vi "Main Tclk.vi"() -> ()   [LabVIEW 2018] (continued)
                                n3267 = local write "SEM Scan Parameters"(w8659) -> ()
                                n3268 = Build Array(w8675, w8670) -> (w8655:T76)
                                n3269 = local write "Auto Aln X"(w8655) -> ()
                              }
                            }
                          }
                          frame #2 {
                            n3270 = Array Size(array=w8677) -> (size(s)=w8680:i32)
                            n3271 = Greater Or Equal?(x=w8680, y=2) -> (x >= y?=w8681:bool)
                            n3272 = Array Subset(array=w8678, length=w8680) -> (w8679:sgl[])  [unwired: 1 in]
                            n3273 = case shown="True" w8681 {
                              tunnel: w8677 -> [_ w8693]
                              tunnel: w8679 -> [_ w8689]
                              tunnel: [_ w8683] -> w8676
                              frame False {
                              }
                              frame True {
                                n3274 = Array Max & Min(array=w8689) -> (max value=w8691:sgl, min value=w8690:sgl)  [unwired: 2 out]
                                n3275 = Array Max & Min(array=w8693) -> (max value=w8695:sgl, min value=w8696:sgl)  [unwired: 2 out]
                                n3276 = Subtract(x=w8691, y=w8690) -> (x-y=w8692:sgl)
                                n3277 = Subtract(x=w8695, y=w8696) -> (x-y=w8694:sgl)
                                n3278 = expression code="x*0.2"(w8692) -> (w8688:sgl)
                                n3279 = expression code="x*0.2"(w8694) -> (w8697:sgl)
                                n3280 = Add(x=w8691, y=w8688) -> (x+y=w8687:sgl)
                                n3281 = Subtract(x=w8690, y=w8688) -> (x-y=w8686:sgl)
                                n3282 = Add(x=w8695, y=w8697) -> (x+y=w8685:sgl)
                                n3283 = Subtract(x=w8696, y=w8697) -> (x-y=w8684:sgl)
                                n3284 = Bundle(w8687, w8686, w8685, w8684) -> (w8683:cluster{sgl, sgl, sgl, sgl})  [unwired: 1 in]
                                n3285 = property on="Auto Aln X" class="XYGraph (strict)"("XScale.Maximum"=w8687, "XScale.Minimum"=w8686, "YScale.Maximum"=w8685, "YScale.Minimum"=w8684) -> ()  [unwired: 2 in, 2 out]
                              }
                            }
                          }
                        }
                      }
                    }
                    n3286 = And Array Elements(Boolean array=w8539) -> (logical AND=w8538:bool)
                    n3287 = local write "AAX Success tiled"(w8541) -> ()
                    n3288 = local write "AAX Graph scales tiled"(w8536) -> ()
                    n3289 = local write "AlnX array tiled"(w8545) -> ()
                    n3290 = local write "AAX Graph tiled"(w8537) -> ()
                    n3291 = local write "Best Aln X FI tiled"(w8543) -> ()
                    n3292 = local write "Skip Steps tiled"(w8544) -> ()
                    n3293 = local write "Best Aln X (%) tiled"(w8542) -> ()
                    n3294 = case shown="True" w8538 {
                      frame False {
                      }
                      frame True {
                        w8557 = T44."Enabled" ("Disabled")
                        w8559 = sgl[][][] [] ("FI array tiled")
                        n3295 = local read "SEM Scan Parameters"() -> (w8556:T26)
                        n3296 = Unbundle By Name(w8556) -> ("Y tiles"=w8552:u8, "X tiles"=w8553:u8)
                        n3297 = local write "AA Count"(u8 0 ("AA Count")) -> ()
                        n3298 = local write "FI array tiled"(w8559) -> ()
                        n3299 = local write "AlnX array tiled"(w8559) -> ()
                        n3300 = local write "Aln Options"(enum16{"Defaut", "Aln X", "Aln Y"}."Aln Y" ("Aln Options")) -> ()
                        n3301 = property on="Auto Align" class="Bool (strict)"("DisabledEnum"=w8557) -> ()  [unwired: 2 in, 2 out]
                        n3302 = property on="AA Steps" class="DigNum (strict)"("DisabledEnum"=w8557) -> ()  [unwired: 2 in, 2 out]
                        n3303 = Initialize Array(u8 0 ("Skip Steps"), w8552, w8553) -> (w8554:u8[][])
                        n3304 = local write "Skip Steps tiled"(w8554) -> ()
                      }
                    }
                  }
                  frame True {
                  }
                }
              }
              frame #35 {
                n3305 = local read "AlnY array tiled"() -> (w8699:sgl[][][])
                n3306 = local read "FI array tiled"() -> (w8700:sgl[][][])
                n3307 = local read "AA Count"() -> (w8701:u8)
                n3308 = local read "AA Steps"() -> (w8703:u8)
                n3309 = local read "Skip Steps tiled"() -> (w8702:u8[][])
                n3310 = local read "Auto Align"() -> (w8704:bool)
                n3311 = Empty Array?(array=w8699) -> (empty?=w8698:bool)
                n3312 = Not(x=w8704) -> (.not. x?=w8705:bool)
                n3313 = case shown="False" w8698 {
                  tunnel: w8699 -> [w8720 _]
                  tunnel: w8700 -> [w8719 _]
                  tunnel: w8701 -> [w8718 _]
                  tunnel: w8702 -> [w8717 _]
                  tunnel: w8703 -> [w8716 _]
                  tunnel: w8705 -> [w8710 _]
                  frame False {
                    n3314 = for {
                      tunnel: w8720 -> [w8741] mode=indexing
                      tunnel: w8719 -> [w8740] mode=indexing
                      tunnel: w8718 -> [w8739]
                      tunnel: w8717 -> [w8738] mode=indexing
                      tunnel: w8716 -> [w8737]
                      tunnel: [w8736] -> w8715 mode=indexing
                      tunnel: [w8734] -> w8714 mode=indexing
                      tunnel: [w8733] -> w8713 mode=indexing
                      tunnel: [w8732] -> w8712 mode=indexing
                      tunnel: [w8731] -> w8711 mode=indexing
                      tunnel: w8710 -> [w8730]
                      tunnel: [w8729] -> w8709 mode=indexing
                      tunnel: [w8728] -> w8707 mode=indexing
                      tunnel: [w8727] -> w8706 mode=indexing
                      i -> [w8735]
                      n3315 = for {
                        tunnel: w8741 -> [w8757] mode=indexing
                        tunnel: w8740 -> [w8756] mode=indexing
                        tunnel: w8739 -> [w8755]
                        tunnel: w8738 -> [w8754] mode=indexing
                        tunnel: w8737 -> [w8753]
                        tunnel: [w8752] -> w8736 mode=indexing
                        tunnel: w8735 -> [w8751]
                        tunnel: [w8749] -> w8734 mode=indexing
                        tunnel: [w8748] -> w8733 mode=indexing
                        tunnel: [w8747] -> w8732 mode=indexing
                        tunnel: [w8746] -> w8731 mode=indexing
                        tunnel: w8730 -> [w8745]
                        tunnel: [w8744] -> w8729 mode=indexing
                        tunnel: [w8743] -> w8728 mode=indexing
                        tunnel: [w8742] -> w8727 mode=indexing
                        i -> [w8750]
                        n3316 = stacked-sequence {
                          seq-local: [w8760 _ _] -> [_ w8798 _]
                          seq-local: [w8758 _ _] -> [_ w8789 _]
                          tunnel: w8757 -> [w8765 w8790 w8845]
                          tunnel: w8756 -> [w8764 w8803 w8844]
                          tunnel: w8755 -> [w8762 w8786 _]
                          tunnel: w8754 -> [w8759 _ _]
                          tunnel: w8753 -> [w8761 w8787 _]
                          tunnel: [_ w8799 _] -> w8752
                          tunnel: w8751 -> [_ w8797 _]
                          tunnel: w8750 -> [_ w8796 _]
                          tunnel: [w8758 _ _] -> w8749
                          tunnel: [_ w8795 _] -> w8748
                          tunnel: [_ w8794 _] -> w8747
                          tunnel: [_ w8793 _] -> w8746
                          tunnel: w8745 -> [_ w8792 _]
                          tunnel: [_ w8791 _] -> w8744
                          tunnel: [_ w8788 _] -> w8743
                          tunnel: [_ _ w8843] -> w8742
                          frame #0 {
                            n3317 = Subtract(x=w8761, y=w8759) -> (x-y=w8763:u8)
                            n3318 = Less?(x=w8762, y=w8763) -> (x < y?=w8766:bool)
                            n3319 = case shown="True" w8766 {
                              tunnel: w8765 -> [w8768 w8773]
                              tunnel: w8762 -> [_ w8772]
                              tunnel: w8764 -> [_ w8774]
                              tunnel: [w8768 w8771] -> w8760
                              tunnel: w8759 -> [w8767 w8770]
                              tunnel: [w8767 w8769] -> w8758
                              frame False {
                              }
                              frame True {
                                n3320 = Index Array(array=w8773, index=w8772) -> (element=w8776:sgl)
                                n3321 = call "1D Parabolic Max.vi"("Y"=w8774, "Xt"=w8776, "X"=w8773) -> ("Y(Xt) < Ymin"=w8775:bool)  [unwired: 1 in, 7 out]
                                n3322 = case shown="True" w8775 {
                                tunnel: w8772 -> [_ w8782]
                                tunnel: w8773 -> [w8778 w8783]
                                tunnel: w8770 -> [w8777 w8780]
                                tunnel: [w8778 w8781] -> w8771
                                tunnel: [w8777 w8779] -> w8769
                                frame False {
                                }
                                frame True {
                                n3323 = Delete From Array(array=w8783, length=1, index=w8782) -> (array with subset deleted=w8781:sgl[])  [unwired: 1 out]
                                n3324 = Increment(x=w8780) -> (x+1=w8779:u8)
                                }
                                }
                              }
                            }
                          }
                          frame #1 {
                            n3325 = Subtract(x=w8787, y=w8789) -> (x-y=w8802:u8)
                            n3326 = call "1D Parabolic Max.vi"("Y"=w8803, "X"=w8790) -> ("Found max"=w8793:bool, "Ymax"=w8800:dbl, "Xmax"=w8804:dbl, "Finer Best Polynomial Fit"=w8806:dbl[], "Finer X"=w8801:dbl[])  [unwired: 2 in, 3 out]
                            n3327 = Greater Or Equal?(x=w8786, y=w8802) -> (x >= y?=w8805:bool)
                            n3328 = Subtract(x=w8787, y=w8786) -> (x-y=w8785:u8)
                            n3329 = Compound Arithmetic op=OR(w8793, w8805, w8792) -> (w8791:bool)
                            n3330 = case shown="True" w8791 {
                              tunnel: w8804 -> [_ w8824]
                              tunnel: w8803 -> [w8808 w8836]
                              tunnel: w8798 -> [w8816 _]
                              tunnel: w8806 -> [_ w8835]
                              tunnel: w8801 -> [_ w8834]
                              tunnel: w8800 -> [_ w8825]
                              tunnel: w8785 -> [_ w8833]
                              tunnel: w8786 -> [_ w8831]
                              tunnel: [w8816 w8830] -> w8799
                              tunnel: w8797 -> [w8813 w8821]
                              tunnel: w8796 -> [w8814 w8820]
                              tunnel: [w8807 w8825] -> w8795
                              tunnel: [w8810 w8824] -> w8794
                              tunnel: w8790 -> [w8811 w8823]
                              tunnel: [w8815 w8822] -> w8788
                              frame False {
                                n3331 = Build Cluster Array(w8811, w8808) -> (w8817:cluster{"Center":sgl, "A Img Focus Index":sgl}[])
                                n3332 = Sort 1D Array(array=w8817) -> (sorted array=w8818:cluster{"Center":sgl, "A Img Focus Index":sgl}[])
                                n3333 = Bundle(w8818) -> (w8819:T74)  [unwired: 1 in]
                                n3334 = Build Array(w8819) -> (w8815:T75)
                                n3335 = local write "AAY Y tile"(w8813) -> ()
                                n3336 = local write "AAY X tile"(w8814) -> ()
                                n3337 = local write "Auto Aln Y"(w8815) -> ()
                                n3338 = Index Array(array=w8811, index=0) -> (element=w8810:sgl)
                                n3339 = Index Array(array=w8808, index=0) -> (element=w8807:sgl)
                              }
                              frame True {
                                n3340 = local read "SEM Scan Parameters"() -> (w8828:T26)
                                n3341 = Initialize Array(w8824, w8833) -> (w8832:dbl[])
                                n3342 = Replace Array Subset(array=w8823, new element=w8832, index=w8831) -> (w8830:sgl[])
                                n3343 = Build Cluster Array(w8823, w8836) -> (w8841:cluster{"Center":sgl, "A Img Focus Index":sgl}[])
                                n3344 = Build Cluster Array(w8834, w8835) -> (w8838:cluster{dbl, dbl}[])
                                n3345 = local write "AAY Y tile"(w8821) -> ()
                                n3346 = local write "AAY X tile"(w8820) -> ()
                                n3347 = Unbundle By Name(w8828) -> ("Y aln"=w8829:sgl[][])
                                n3348 = Sort 1D Array(array=w8841) -> (sorted array=w8840:cluster{"Center":sgl, "A Img Focus Index":sgl}[])
                                n3349 = Sort 1D Array(array=w8838) -> (sorted array=w8839:cluster{dbl, dbl}[])
                                n3350 = Replace Array Subset(array=w8829, new element=w8824, index (row)=w8821, index (col)=w8820) -> (w8827:sgl[][])
                                n3351 = Bundle(w8840) -> (w8842:T74)  [unwired: 1 in]
                                n3352 = Bundle(w8839) -> (w8837:cluster{cluster{dbl, dbl}[]})  [unwired: 1 in]
                                n3353 = Bundle By Name(cluster=w8828, "Y aln"=w8827) -> (w8826:T26)
                                n3354 = local write "SEM Scan Parameters"(w8826) -> ()
                                n3355 = Build Array(w8842, w8837) -> (w8822:T76)
                                n3356 = local write "Auto Aln Y"(w8822) -> ()
                              }
                            }
                          }
                          frame #2 {
                            n3357 = Array Size(array=w8844) -> (size(s)=w8847:i32)
                            n3358 = Greater Or Equal?(x=w8847, y=2) -> (x >= y?=w8848:bool)
                            n3359 = Array Subset(array=w8845, length=w8847) -> (w8846:sgl[])  [unwired: 1 in]
                            n3360 = case shown="True" w8848 {
                              tunnel: w8844 -> [_ w8860]
                              tunnel: w8846 -> [_ w8856]
                              tunnel: [_ w8850] -> w8843
                              frame False {
                              }
                              frame True {
                                n3361 = Array Max & Min(array=w8856) -> (max value=w8858:sgl, min value=w8857:sgl)  [unwired: 2 out]
                                n3362 = Array Max & Min(array=w8860) -> (max value=w8862:sgl, min value=w8863:sgl)  [unwired: 2 out]
                                n3363 = Subtract(x=w8858, y=w8857) -> (x-y=w8859:sgl)
                                n3364 = Subtract(x=w8862, y=w8863) -> (x-y=w8861:sgl)
                                n3365 = expression code="x*0.2"(w8859) -> (w8855:sgl)
                                n3366 = expression code="x*0.2"(w8861) -> (w8864:sgl)
                                n3367 = Add(x=w8858, y=w8855) -> (x+y=w8854:sgl)
                                n3368 = Subtract(x=w8857, y=w8855) -> (x-y=w8853:sgl)
                                n3369 = Add(x=w8862, y=w8864) -> (x+y=w8852:sgl)
                                n3370 = Subtract(x=w8863, y=w8864) -> (x-y=w8851:sgl)
                                n3371 = Bundle(w8854, w8853, w8852, w8851) -> (w8850:cluster{sgl, sgl, sgl, sgl})  [unwired: 1 in]
                                n3372 = property on="Auto Aln Y" class="XYGraph (strict)"("XScale.Maximum"=w8854, "XScale.Minimum"=w8853, "YScale.Maximum"=w8852, "YScale.Minimum"=w8851) -> ()  [unwired: 2 in, 2 out]
                              }
                            }
                          }
                        }
                      }
                    }
                    n3373 = And Array Elements(Boolean array=w8709) -> (logical AND=w8708:bool)
                    n3374 = local write "AAY Success tiled"(w8711) -> ()
                    n3375 = local write "AAY Graph scales tiled"(w8706) -> ()
                    n3376 = local write "AlnY array tiled"(w8715) -> ()
                    n3377 = local write "AAY Graph tiled"(w8707) -> ()
                    n3378 = local write "Best Aln Y FI tiled"(w8713) -> ()
                    n3379 = local write "Skip Steps tiled"(w8714) -> ()
                    n3380 = local write "Best Aln Y (%) tiled"(w8712) -> ()
                    n3381 = case shown="True" w8708 {
                      frame False {
                      }
                      frame True {
                        w8723 = T44."Enabled" ("Disabled")
                        w8725 = sgl[][][] [] ("FI array tiled")
                        n3382 = local write "Auto Align"(FALSE ("Auto Stig")) -> ()
                        n3383 = local write "AA Count"(u8 0 ("AA Count")) -> ()
                        n3384 = local write "Skip Steps tiled"(u8[][] [] ("AS Count tiled")) -> ()
                        n3385 = local write "FI array tiled"(w8725) -> ()
                        n3386 = local write "AlnX array tiled"(w8725) -> ()
                        n3387 = local write "Aln Options"(enum16{"Defaut", "Aln X", "Aln Y"}."Defaut" ("Aln Options")) -> ()
                        n3388 = property on="Auto Focus" class="Bool (strict)"("DisabledEnum"=w8723) -> ()  [unwired: 2 in, 2 out]
                        n3389 = property on="Auto Stig" class="Bool (strict)"("DisabledEnum"=w8723) -> ()  [unwired: 2 in, 2 out]
                        n3390 = property on="Auto Align" class="Bool (strict)"("DisabledEnum"=w8723) -> ()  [unwired: 2 in, 2 out]
                        n3391 = property on="AA Steps" class="DigNum (strict)"("DisabledEnum"=w8723) -> ()  [unwired: 2 in, 2 out]
                      }
                    }
                  }
                  frame True {
                  }
                }
              }
              frame #36 {
                n3392 = local read "Low Mag SEM"() -> (w8865:T30)
                n3393 = local read "Mid Mag SEM"() -> (w8866:T29)
                n3394 = Unbundle By Name(w8865) -> ("Low mag scan"=w8867:bool)
                n3395 = Unbundle By Name(w8866) -> ("Mid mag scan"=w8868:bool)
                n3396 = case shown="True" w8867 {
                  tunnel: w8865 -> [_ w8891]
                  frame False {
                  }
                  frame True {
                    w8887 = sgl[] [0.0] ("dX (um)")
                    w8888 = u8 1 ("X tiles")
                    w8892 = 0.0 ("X center")
                    n3397 = Unbundle By Name(w8891) -> ("Low mag scan FOV (micron)"=w8889:dbl, "Low mag scan rate (Hz)"=w8901:u32)
                    n3398 = local read "SEM Scan Parameters"() -> (w8894:T26)
                    n3399 = Unbundle By Name(w8894) -> ("Scan rate (Hz)"=w8896:u32, "Oversampling"=w8895:u32)
                    n3400 = expression code="x*1000"(w8889) -> (w8902:dbl)
                    n3401 = Multiply(x=w8896, y=w8895) -> (x*y=w8897:u32)
                    n3402 = Divide(x=w8897, y=w8901) -> (x/y=w8898:dbl)
                    n3403 = Divide(x=w8902, y=u32 512 ("X resolution")) -> (x/y=w8900:dbl)
                    n3404 = Bundle By Name(cluster=w8894, "X size (um)"=w8889, "Y size (um)"=w8889, "X center (um)"=w8892, "Y center (um)"=w8892, "X size (V)"=20.0, "Scan rate (Hz)"=w8901, "Oversampling"=w8898, "X tiles"=w8888, "Y tiles"=w8888, "Frames"=w8888, "dX (um)"=w8887, "dY (um)"=w8887, "Pixel size (nm)"=w8900) -> (w8890:T26)
                    n3405 = local write "SEM Low Mag Scan Parameters"(w8890) -> ()
                  }
                }
                n3406 = case shown="True" w8868 {
                  tunnel: w8866 -> [_ w8875]
                  frame False {
                  }
                  frame True {
                    w8869 = sgl[] [0.0] ("dX (um)")
                    w8870 = u8 1 ("X tiles")
                    n3407 = Unbundle By Name(w8875) -> ("X size (um)"=w8881:sgl, "Y size (um)"=w8880:sgl, "X center (um)"=w8879:dbl, "Y center (um)"=w8878:dbl, "Mid mag scan rate (Hz)"=w8877:u32, "Pixel size (nm)"=w8876:sgl)
                    n3408 = local read "SEM Mid Mag Scan Parameters"() -> (w8873:T5)
                    n3409 = local read "SEM Scan Parameters"() -> (w8882:T26)
                    n3410 = Unbundle By Name(w8882) -> ("Scan rate (Hz)"=w8884:u32, "Oversampling"=w8883:u32)
                    n3411 = Unbundle By Name(w8873) -> ("X size (V)"=w8872:dbl)
                    n3412 = Multiply(x=w8884, y=w8883) -> (x*y=w8885:u32)
                    n3413 = Divide(x=w8885, y=w8877) -> (x/y=w8886:dbl)
                    n3414 = Bundle By Name(cluster=w8882, "X size (um)"=w8881, "Y size (um)"=w8880, "X center (um)"=w8879, "Y center (um)"=w8878, "Oversampling auto"=TRUE ("X size auto"), "Scan rate (Hz)"=w8877, "Oversampling"=w8886, "Pixel size (nm)"=w8876, "X size (V)"=w8872, "X tiles"=w8870, "Y tiles"=w8870, "Frames"=w8870, "dX (um)"=w8869, "dY (um)"=w8869) -> (w8871:T26)
                    n3415 = local write "SEM Mid Mag Scan Parameters"(w8871) -> ()
                  }
                }
              }
              frame #37 {
                n3416 = local read "Mid Mag SEM"() -> (w8917:T29)
                n3417 = local read "FIB slice #"() -> (w8911:u32)
                n3418 = Unbundle By Name(w8917) -> ("Mid mag scan"=w8918:bool, "Prior to main scan"=w8919:bool, "Mid mag interval"=w8905:u32)
                n3419 = Equal?(x=u32 1 ("y"), y=w8905) -> (x = y?=w8909:bool)
                n3420 = case shown="False" w8909 {
                  tunnel: [w8923 w8926] -> w8907
                  tunnel: [w8922 w8926] -> w8908
                  tunnel: [w8920 w8926] -> w8906
                  frame False {
                    n3421 = local read "Auto Focus"() -> (w8925:bool)
                    n3422 = local read "Auto Stig"() -> (w8924:bool)
                    n3423 = local read "Auto Align"() -> (w8921:bool)
                    n3424 = Not(x=w8925) -> (.not. x?=w8922:bool)
                    n3425 = Not(x=w8924) -> (.not. x?=w8923:bool)
                    n3426 = Not(x=w8921) -> (.not. x?=w8920:bool)
                  }
                  frame True {
                    w8926 = TRUE
                  }
                }
                n3427 = Subtract(x=w8911, y=u32 2) -> (x-y=w8903:u32)
                n3428 = Quotient & Remainder(x=w8903, y=w8905) -> (x-y*floor(x/y)=w8915:u32)  [unwired: 1 out]
                n3429 = local read "FIB"() -> (w8912:bool)
                n3430 = Not(x=w8919) -> (.not. x?=w8914:bool)
                n3431 = Equal To 0?(x=w8915) -> (x = 0?=w8916:bool)
                n3432 = Compound Arithmetic op=AND(w8912, w8908, w8907, w8906, w8918, w8914, w8916) -> (w8913:bool)
                n3433 = case shown="True" w8913 {
                  frame False {
                    n3434 = local write "Mid Mag SEM on"(FALSE ("Mid Mag SEM on")) -> ()
                    n3435 = local write "MM overhead"(u32 0 ("MM overhead")) -> ()
                  }
                  frame True {
                    w8938 = FALSE ("GetInfo")
                    n3436 = local read "Tiled scan inputs"() -> (w8937:T6)
                    n3437 = local read "SEM Mid Mag Scan Parameters"() -> (w8935:T5)
                    n3438 = local read "File Information"() -> (w8934:T31)
                    n3439 = local write "Mid Mag SEM on"(TRUE ("Mid Mag SEM on")) -> ()
                    n3440 = Unbundle By Name(w8934) -> ("File path"=w8932:path)
                    n3441 = local write "Status message"("SEM Mid Mag Scan" ("Status message")) -> ()
                    n3442 = local read "MM SEM scan time"() -> (w8929:dbl)
                    n3443 = Build Path(base path=w8932, name or relative path="Mid Mag Scans\\") -> (appended path=w8931:path)
                    n3444 = Bundle By Name(cluster=w8937, "SEM Options.GetInfo"=w8938, "SEM Options.PNG only"=w8938, "SEM Options.Upload"=w8938, "SEM Scan Parameters"=w8935, "File Information.File path"=w8931) -> (w8936:T6)
                    n3445 = expression code="x+10"(w8929) -> (w8930:dbl)
                    n3446 = local write "MM overhead"(w8930) -> ()
                    n3447 = call "2D scan tiled.vi"("Tiled scan inputs"=w8936) -> ()  [unwired: 5 in, 6 out]
                  }
                }
              }
              frame #38 {
                n3448 = local read "Low Mag SEM"() -> (w8946:T30)
                n3449 = local read "FIB slice #"() -> (w8941:u32)
                n3450 = Unbundle By Name(w8946) -> ("Low mag scan"=w8945:bool, "Prior to main scan"=w8944:bool, "Low mag interval"=w8942:u32)
                n3451 = Quotient & Remainder(x=w8941, y=w8942) -> (x-y*floor(x/y)=w8948:u32)  [unwired: 1 out]
                n3452 = local read "FIB"() -> (w8943:bool)
                n3453 = Not(x=w8944) -> (.not. x?=w8949:bool)
                n3454 = Equal To 0?(x=w8948) -> (x = 0?=w8947:bool)
                n3455 = Compound Arithmetic op=AND(w8943, w8945, w8949, w8947) -> (w8950:bool)
                n3456 = case shown="True" w8950 {
                  frame False {
                    n3457 = local write "Low Mag SEM on"(FALSE ("Mid Mag SEM on")) -> ()
                    n3458 = local write "LM overhead"(u32 0 ("LM overhead")) -> ()
                  }
                  frame True {
                    w8957 = FALSE ("GetInfo")
                    n3459 = local read "LM SEM scan time"() -> (w8953:dbl)
                    n3460 = local read "Tiled scan inputs"() -> (w8956:T6)
                    n3461 = local read "SEM Low Mag Scan Parameters"() -> (w8960:T5)
                    n3462 = local read "File Information"() -> (w8961:T31)
                    n3463 = local write "Low Mag SEM on"(TRUE ("Mid Mag SEM on")) -> ()
                    n3464 = Unbundle By Name(w8961) -> ("File path"=w8963:path)
                    n3465 = local write "Status message"("SEM Low Mag Scan" ("Status message")) -> ()
                    n3466 = expression code="x+10"(w8953) -> (w8954:dbl)
                    n3467 = local write "LM overhead"(w8954) -> ()
                    n3468 = Build Path(base path=w8963, name or relative path="Low Mag Scans\\") -> (appended path=w8964:path)
                    n3469 = Bundle By Name(cluster=w8956, "SEM Options.GetInfo"=w8957, "SEM Options.PNG only"=TRUE ("PNG only"), "SEM Options.Upload"=w8957, "SEM Scan Parameters"=w8960, "File Information.File path"=w8964) -> (w8959:T6)
                    n3470 = call "2D scan tiled.vi"("Tiled scan inputs"=w8959) -> ()  [unwired: 5 in, 6 out]
                  }
                }
              }
              frame #39 {
                n3471 = local read "Low Mag SEM"() -> (w8979:T30)
                n3472 = local read "FIB slice #"() -> (w8976:u32)
                n3473 = local read "FIB HW Config"() -> (w8982:T23)
                n3474 = Unbundle By Name(w8979) -> ("Low mag scan"=w8978:bool, "Low mag interval"=w8977:u32)
                n3475 = Unbundle By Name(w8982) -> ("Beam blank"=w8983:tag)
                n3476 = local read "Api"() -> (w8966:refnum<k7>)
                n3477 = Quotient & Remainder(x=w8976, y=w8977) -> (x-y*floor(x/y)=w8981:u32)  [unwired: 1 out]
                n3478 = call "FIB beam blank.vi"("Api"=w8966, "Beam blanked"=TRUE, "lines"=w8983) -> ()  [unwired: 2 in, 1 out]
                n3479 = Equal To 0?(x=w8981) -> (x = 0?=w8980:bool)
                n3480 = Compound Arithmetic op=AND(w8978, w8980) -> (w8975:bool)
                n3481 = local read "Last FIB recipe"() -> (w8971:path)
                n3482 = case shown="True" w8975 {
                  frame False {
                  }
                  frame True {
                    n3483 = local read "FIB Image"() -> (w8996:i16[][])
                    n3484 = Array Size(array=w8996) -> (size(s)=w8997:i32[])
                    n3485 = local read "Pre Image"() -> (w9003:i16[][])
                    n3486 = Array Size(array=w9003) -> (size(s)=w9002:i32[])
                    n3487 = Add Array Elements(numeric array=w8997) -> (sum=w8998:i32)
                    n3488 = Add Array Elements(numeric array=w9002) -> (sum=w9001:i32)
                    n3489 = Not Equal To 0?(x=w8998) -> (x != 0?=w8999:bool)
                    n3490 = Not Equal To 0?(x=w9001) -> (x != 0?=w9000:bool)
                    n3491 = case shown="True" w8999 {
                      tunnel: w8996 -> [_ w9023]
                      frame False {
                      }
                      frame True {
                        n3492 = local read "Last FIB image"() -> (w9026:path)
                        n3493 = call "16bit Image Normalization.vi"("Transpose"=FALSE, "Input image"=w9023) -> ("Normalized image"=w9022:u8[][])  [unwired: 5 in, 4 out]
                        n3494 = call <vilib>:"Flatten Pixmap.vi"("colors"=u32[] [16777222, 65793, 131586, 197379, 263172, 328965, 394758, 460551, 526344, 592137, 657930, 723723, 789516, 855309, 921102, 986895, 1052688, 1118481, 1184274, 1250067, 1315860, 1381653, 1447446, 1513239, 1579032, 1644825, 1710618, 1776411, 1842204, 1907997, 1973790, 2039583, 2105376, 2171169, 2236962, 2302755, 2368548, 2434341, 2500134, 2565927, 2631720, 2697513, 2763306, 2829099, 2894892, 2960685, 3026478, 3092271, 3158064, 3223857, 3289650, 3355443, 3421236, 3487029, 3552822, 3618615, 3684408, 3750201, 3815994, 3881787, 3947580, 4013373, 4079166, 4144959, 4210752, 4276545, 4342338, 4408131, 4473924, 4539717, 4605510, 4671303, 4737096, 4802889, 4868682, 4934475, 5000268, 5066061, 5131854, 5197647, 5263440, 5329233, 5395026, 5460819, 5526612, 5592405, 5658198, 5723991, 5789784, 5855577, 5921370, 5987163, 6052956, 6118749, 6184542, 6250335, 6316128, 6381921, 6447714, 6513507, 6579300, 6645093, 6710886, 6776679, 6842472, 6908265, 6974058, 7039851, 7105644, 7171437, 7237230, 7303023, 7368816, 7434609, 7500402, 7566195, 7631988, 7697781, 7763574, 7829367, 7895160, 7960953, 8026746, 8092539, 8158332, 8224125, 8289918, 8355711, 8421504, 8487297, 8553090, 8618883, 8684676, 8750469, 8816262, 8882055, 8947848, 9013641, 9079434, 9145227, 9211020, 9276813, 9342606, 9408399, 9474192, 9539985, 9605778, 9671571, 9737364, 9803157, 9868950, 9934743, 10000536, 10066329, 10132122, 10197915, 10263708, 10329501, 10395294, 10461087, 10526880, 10592673, 10658466, 10724259, 10790052, 10855845, 10921638, 10987431, 11053224, 11119017, 11184810, 11250603, 11316396, 11382189, 11447982, 11513775, 11579568, 11645361, 11711154, 11776947, 11842740, 11908533, 11974326, 12040119, 12105912, 12171705, 12237498, 12303291, 12369084, 12434877, 12500670, 12566463, 12632256, 12698049, 12763842, 12829635, 12895428, 12961221, 13027014, 13092807, 13158600, 13224393, 13290186, 13355979, 13421772, 13487565, 13553358, 13619151, 13684944, 13750737, 13816530, 13882323, 13948116, 14013909, 14079702, 14145495, 14211288, 14277081, 14342874, 14408667, 14474460, 14540253, 14606046, 14671839, 14737632, 14803425, 14869218, 14935011, 15000804, 15066597, 15132390, 15198183, 15263976, 15329769, 15395562, 15461355, 15527148, 15592941, 15658734, 15724527, 15790320, 15856113, 15921906, 15987699, 16053492, 16119285, 16185078, 16250871, 16316664, 16382457, 16448250, 16514043, 16579836, 16645629, 16711422, 16448250] ("256 gray scale"), "8-bit pixmap"=w9022) -> ("image data"=w9025:T55)  [unwired: 4 in, 5 out]
                        n3495 = call <vilib>:"Write PNG File.vi"("image data"=w9025, "path to PNG file"=w9026) -> ()  [unwired: 1 in, 9 out]
                      }
                    }
                    n3496 = case shown="True" w9000 {
                      tunnel: w9003 -> [_ w9017]
                      frame False {
                      }
                      frame True {
                        n3497 = local read "Last FIB zoom pre image"() -> (w9020:path)
                        n3498 = call "16bit Image Normalization.vi"("Transpose"=FALSE, "Input image"=w9017) -> ("Normalized image"=w9016:u8[][])  [unwired: 5 in, 4 out]
                        n3499 = call <vilib>:"Flatten Pixmap.vi"("colors"=u32[] [16777222, 65793, 131586, 197379, 263172, 328965, 394758, 460551, 526344, 592137, 657930, 723723, 789516, 855309, 921102, 986895, 1052688, 1118481, 1184274, 1250067, 1315860, 1381653, 1447446, 1513239, 1579032, 1644825, 1710618, 1776411, 1842204, 1907997, 1973790, 2039583, 2105376, 2171169, 2236962, 2302755, 2368548, 2434341, 2500134, 2565927, 2631720, 2697513, 2763306, 2829099, 2894892, 2960685, 3026478, 3092271, 3158064, 3223857, 3289650, 3355443, 3421236, 3487029, 3552822, 3618615, 3684408, 3750201, 3815994, 3881787, 3947580, 4013373, 4079166, 4144959, 4210752, 4276545, 4342338, 4408131, 4473924, 4539717, 4605510, 4671303, 4737096, 4802889, 4868682, 4934475, 5000268, 5066061, 5131854, 5197647, 5263440, 5329233, 5395026, 5460819, 5526612, 5592405, 5658198, 5723991, 5789784, 5855577, 5921370, 5987163, 6052956, 6118749, 6184542, 6250335, 6316128, 6381921, 6447714, 6513507, 6579300, 6645093, 6710886, 6776679, 6842472, 6908265, 6974058, 7039851, 7105644, 7171437, 7237230, 7303023, 7368816, 7434609, 7500402, 7566195, 7631988, 7697781, 7763574, 7829367, 7895160, 7960953, 8026746, 8092539, 8158332, 8224125, 8289918, 8355711, 8421504, 8487297, 8553090, 8618883, 8684676, 8750469, 8816262, 8882055, 8947848, 9013641, 9079434, 9145227, 9211020, 9276813, 9342606, 9408399, 9474192, 9539985, 9605778, 9671571, 9737364, 9803157, 9868950, 9934743, 10000536, 10066329, 10132122, 10197915, 10263708, 10329501, 10395294, 10461087, 10526880, 10592673, 10658466, 10724259, 10790052, 10855845, 10921638, 10987431, 11053224, 11119017, 11184810, 11250603, 11316396, 11382189, 11447982, 11513775, 11579568, 11645361, 11711154, 11776947, 11842740, 11908533, 11974326, 12040119, 12105912, 12171705, 12237498, 12303291, 12369084, 12434877, 12500670, 12566463, 12632256, 12698049, 12763842, 12829635, 12895428, 12961221, 13027014, 13092807, 13158600, 13224393, 13290186, 13355979, 13421772, 13487565, 13553358, 13619151, 13684944, 13750737, 13816530, 13882323, 13948116, 14013909, 14079702, 14145495, 14211288, 14277081, 14342874, 14408667, 14474460, 14540253, 14606046, 14671839, 14737632, 14803425, 14869218, 14935011, 15000804, 15066597, 15132390, 15198183, 15263976, 15329769, 15395562, 15461355, 15527148, 15592941, 15658734, 15724527, 15790320, 15856113, 15921906, 15987699, 16053492, 16119285, 16185078, 16250871, 16316664, 16382457, 16448250, 16514043, 16579836, 16645629, 16711422, 16448250] ("256 gray scale"), "8-bit pixmap"=w9016) -> ("image data"=w9019:T55)  [unwired: 4 in, 5 out]
                        n3500 = call <vilib>:"Write PNG File.vi"("image data"=w9019, "path to PNG file"=w9020) -> ()  [unwired: 1 in, 9 out]
                      }
                    }
                    n3501 = local read "Detector A Low Mag"() -> (w8994:i16[][])
                    n3502 = local read "Detector B Low Mag"() -> (w8995:i16[][])
                    n3503 = Array Size(array=w8994) -> (size(s)=w8993:i32[])
                    n3504 = Array Size(array=w8995) -> (size(s)=w8988:i32[])
                    n3505 = Add Array Elements(numeric array=w8993) -> (sum=w8992:i32)
                    n3506 = Add Array Elements(numeric array=w8988) -> (sum=w8989:i32)
                    n3507 = Not Equal To 0?(x=w8992) -> (x != 0?=w8991:bool)
                    n3508 = Not Equal To 0?(x=w8989) -> (x != 0?=w8990:bool)
                    n3509 = case shown="True" w8991 {
                      tunnel: w8994 -> [_ w9011]
                      frame False {
                      }
                      frame True {
                        n3510 = local read "Last Det A Low Mag"() -> (w9014:path)
                        n3511 = call "16bit Image Normalization.vi"("Transpose"=FALSE, "Input image"=w9011) -> ("Normalized image"=w9010:u8[][])  [unwired: 5 in, 4 out]
                        n3512 = call <vilib>:"Flatten Pixmap.vi"("colors"=u32[] [16777222, 65793, 131586, 197379, 263172, 328965, 394758, 460551, 526344, 592137, 657930, 723723, 789516, 855309, 921102, 986895, 1052688, 1118481, 1184274, 1250067, 1315860, 1381653, 1447446, 1513239, 1579032, 1644825, 1710618, 1776411, 1842204, 1907997, 1973790, 2039583, 2105376, 2171169, 2236962, 2302755, 2368548, 2434341, 2500134, 2565927, 2631720, 2697513, 2763306, 2829099, 2894892, 2960685, 3026478, 3092271, 3158064, 3223857, 3289650, 3355443, 3421236, 3487029, 3552822, 3618615, 3684408, 3750201, 3815994, 3881787, 3947580, 4013373, 4079166, 4144959, 4210752, 4276545, 4342338, 4408131, 4473924, 4539717, 4605510, 4671303, 4737096, 4802889, 4868682, 4934475, 5000268, 5066061, 5131854, 5197647, 5263440, 5329233, 5395026, 5460819, 5526612, 5592405, 5658198, 5723991, 5789784, 5855577, 5921370, 5987163, 6052956, 6118749, 6184542, 6250335, 6316128, 6381921, 6447714, 6513507, 6579300, 6645093, 6710886, 6776679, 6842472, 6908265, 6974058, 7039851, 7105644, 7171437, 7237230, 7303023, 7368816, 7434609, 7500402, 7566195, 7631988, 7697781, 7763574, 7829367, 7895160, 7960953, 8026746, 8092539, 8158332, 8224125, 8289918, 8355711, 8421504, 8487297, 8553090, 8618883, 8684676, 8750469, 8816262, 8882055, 8947848, 9013641, 9079434, 9145227, 9211020, 9276813, 9342606, 9408399, 9474192, 9539985, 9605778, 9671571, 9737364, 9803157, 9868950, 9934743, 10000536, 10066329, 10132122, 10197915, 10263708, 10329501, 10395294, 10461087, 10526880, 10592673, 10658466, 10724259, 10790052, 10855845, 10921638, 10987431, 11053224, 11119017, 11184810, 11250603, 11316396, 11382189, 11447982, 11513775, 11579568, 11645361, 11711154, 11776947, 11842740, 11908533, 11974326, 12040119, 12105912, 12171705, 12237498, 12303291, 12369084, 12434877, 12500670, 12566463, 12632256, 12698049, 12763842, 12829635, 12895428, 12961221, 13027014, 13092807, 13158600, 13224393, 13290186, 13355979, 13421772, 13487565, 13553358, 13619151, 13684944, 13750737, 13816530, 13882323, 13948116, 14013909, 14079702, 14145495, 14211288, 14277081, 14342874, 14408667, 14474460, 14540253, 14606046, 14671839, 14737632, 14803425, 14869218, 14935011, 15000804, 15066597, 15132390, 15198183, 15263976, 15329769, 15395562, 15461355, 15527148, 15592941, 15658734, 15724527, 15790320, 15856113, 15921906, 15987699, 16053492, 16119285, 16185078, 16250871, 16316664, 16382457, 16448250, 16514043, 16579836, 16645629, 16711422, 16448250] ("256 gray scale"), "8-bit pixmap"=w9010) -> ("image data"=w9013:T55)  [unwired: 4 in, 5 out]
                        n3513 = call <vilib>:"Write PNG File.vi"("image data"=w9013, "path to PNG file"=w9014) -> ()  [unwired: 1 in, 9 out]
                      }
                    }
                    n3514 = case shown="True" w8990 {
                      tunnel: w8995 -> [_ w9005]
                      frame False {
                      }
                      frame True {
                        n3515 = local read "Last Det B Low Mag"() -> (w9008:path)
                        n3516 = call "16bit Image Normalization.vi"("Transpose"=FALSE, "Input image"=w9005) -> ("Normalized image"=w9004:u8[][])  [unwired: 5 in, 4 out]
                        n3517 = call <vilib>:"Flatten Pixmap.vi"("colors"=u32[] [16777222, 65793, 131586, 197379, 263172, 328965, 394758, 460551, 526344, 592137, 657930, 723723, 789516, 855309, 921102, 986895, 1052688, 1118481, 1184274, 1250067, 1315860, 1381653, 1447446, 1513239, 1579032, 1644825, 1710618, 1776411, 1842204, 1907997, 1973790, 2039583, 2105376, 2171169, 2236962, 2302755, 2368548, 2434341, 2500134, 2565927, 2631720, 2697513, 2763306, 2829099, 2894892, 2960685, 3026478, 3092271, 3158064, 3223857, 3289650, 3355443, 3421236, 3487029, 3552822, 3618615, 3684408, 3750201, 3815994, 3881787, 3947580, 4013373, 4079166, 4144959, 4210752, 4276545, 4342338, 4408131, 4473924, 4539717, 4605510, 4671303, 4737096, 4802889, 4868682, 4934475, 5000268, 5066061, 5131854, 5197647, 5263440, 5329233, 5395026, 5460819, 5526612, 5592405, 5658198, 5723991, 5789784, 5855577, 5921370, 5987163, 6052956, 6118749, 6184542, 6250335, 6316128, 6381921, 6447714, 6513507, 6579300, 6645093, 6710886, 6776679, 6842472, 6908265, 6974058, 7039851, 7105644, 7171437, 7237230, 7303023, 7368816, 7434609, 7500402, 7566195, 7631988, 7697781, 7763574, 7829367, 7895160, 7960953, 8026746, 8092539, 8158332, 8224125, 8289918, 8355711, 8421504, 8487297, 8553090, 8618883, 8684676, 8750469, 8816262, 8882055, 8947848, 9013641, 9079434, 9145227, 9211020, 9276813, 9342606, 9408399, 9474192, 9539985, 9605778, 9671571, 9737364, 9803157, 9868950, 9934743, 10000536, 10066329, 10132122, 10197915, 10263708, 10329501, 10395294, 10461087, 10526880, 10592673, 10658466, 10724259, 10790052, 10855845, 10921638, 10987431, 11053224, 11119017, 11184810, 11250603, 11316396, 11382189, 11447982, 11513775, 11579568, 11645361, 11711154, 11776947, 11842740, 11908533, 11974326, 12040119, 12105912, 12171705, 12237498, 12303291, 12369084, 12434877, 12500670, 12566463, 12632256, 12698049, 12763842, 12829635, 12895428, 12961221, 13027014, 13092807, 13158600, 13224393, 13290186, 13355979, 13421772, 13487565, 13553358, 13619151, 13684944, 13750737, 13816530, 13882323, 13948116, 14013909, 14079702, 14145495, 14211288, 14277081, 14342874, 14408667, 14474460, 14540253, 14606046, 14671839, 14737632, 14803425, 14869218, 14935011, 15000804, 15066597, 15132390, 15198183, 15263976, 15329769, 15395562, 15461355, 15527148, 15592941, 15658734, 15724527, 15790320, 15856113, 15921906, 15987699, 16053492, 16119285, 16185078, 16250871, 16316664, 16382457, 16448250, 16514043, 16579836, 16645629, 16711422, 16448250] ("256 gray scale"), "8-bit pixmap"=w9004) -> ("image data"=w9007:T55)  [unwired: 4 in, 5 out]
                        n3518 = call <vilib>:"Write PNG File.vi"("image data"=w9007, "path to PNG file"=w9008) -> ()  [unwired: 1 in, 9 out]
                      }
                    }
                  }
                }
                n3519 = expression code="x*1000"("SEM-FIB Delay (s)") -> (w8967:u32)
                n3520 = Open/Create/Replace File(file path (use dialog)=w8971) -> (error out=w8973:errorcluster)  [unwired: 5 in, 2 out]
                n3521 = Wait (ms)(milliseconds to wait=w8967) -> ()  [unwired: 1 out]
                n3522 = Unbundle By Name(w8973) -> ("status"=w8972:bool)
                n3523 = local read "Recipe input"() -> (w8969:T7)
                n3524 = case shown="False" w8972 {
                  tunnel: w8971 -> [w8986 w8987]
                  tunnel: [w8985 w8987] -> w8974
                  frame False {
                    n3525 = Delete(path (use dialog)=w8986) -> (deleted path=w8985:path)  [unwired: 4 in, 2 out]
                  }
                  frame True {
                  }
                }
                n3526 = call "Recipe read write.vi"("Write"=TRUE, "Recipe path"=w8974, "Write input"=w8969) -> ()  [unwired: 5 in, 4 out]
              }
              frame #40 {
                n3527 = local read "Alert Settings"() -> (w9079:T36)
                n3528 = local read "Milling para"() -> (w9029:T35)
                n3529 = local read "SEM Scan Parameters"() -> (w9049:T26)
                n3530 = Unbundle By Name(w9049) -> ("Pixel size (nm)"=w9044:sgl)
                n3531 = local read "Temp array"() -> (w9113:sgl[])
                n3532 = local read "Alert Settings"() -> (w9106:T36)
                n3533 = Unbundle By Name(w9029) -> ("FIB PID target"=w9086:sgl, "FIB PID on"=w9091:bool, "FIB PID measured"=w9089:u8)
                n3534 = local read "Milling Z voltage array"() -> (w9084:sgl[])
                n3535 = local read "Auto re-engage"() -> (w9078:bool)
                n3536 = Unbundle By Name(w9079) -> ("Milling Z voltage alarm"=w9064:bool)
                n3537 = local read "FIB"() -> (w9065:bool)
                n3538 = local read "FIB CL control band"() -> (w9028:sgl)
                n3539 = Unbundle By Name(w9029) -> ("FIB PID on"=w9051:bool, "FIB PID measured"=w9050:u8, "FIB PID target"=w9101:sgl, "Lines auto pause"=w9092:u16)
                n3540 = Unbundle By Name(w9106) -> ("Focus index warning"=w9111:bool)
                n3541 = Unbundle By Name(w9029) -> ("Z-step (nm)"=w9093:dbl)
                n3542 = local read "FI below limit counts"() -> (w9112:u8)
                n3543 = Unbundle By Name(w9106) -> ("Focus index stop limit"=w9109:sgl)
                n3544 = Unbundle By Name(w9106) -> ("Temp limit auto"=w9116:bool)
                n3545 = local read "Focus Index"() -> (w9095:sgl)
                n3546 = Array Size(array=w9113) -> (size(s)=w9117:i32)
                n3547 = Not(x=w9078) -> (.not. x?=w9077:bool)
                n3548 = Equal?(x=u8 3, y=w9089) -> (x = y?=w9090:bool)
                n3549 = Compound Arithmetic op=AND(w9077, w9065, w9064) -> (w9076:bool)
                n3550 = In Range and Coerce(upper limit=sgl 50.0, x=w9044, lower limit=sgl 8.0) -> (coerced(x)=w9045:sgl)  [unwired: 1 out]
                n3551 = Greater Or Equal?(x=w9117, y=10 ("x")) -> (x >= y?=w9115:bool)
                n3552 = And(x=w9091, y=w9090) -> (x .and. y?=w9087:bool)
                n3553 = case shown="True" w9076 {
                  tunnel: w9084 -> [_ w9127]
                  tunnel: [FALSE w9120] -> w9080
                  frame False {
                  }
                  frame True {
                    n3554 = call "Auto limits.vi"("Minimum half range"=0.05, "# of interquartile range or stdev"=1.0 ("# of sigma"), "Length"=10, "Input array"=w9127) -> ("Low limit"=w9122:dbl, "High limit"=w9121:dbl)  [unwired: 5 in, 1 out]
                    n3555 = local read "Milling Z voltage (V)"() -> (w9123:sgl)
                    n3556 = In Range and Coerce(upper limit=w9121, x=w9123, lower limit=w9122) -> (In Range?=w9124:bool)  [unwired: 1 out]
                    n3557 = Not(x=w9124) -> (.not. x?=w9120:bool)
                  }
                }
                "Milling Z voltage spike" <- w9080
                n3558 = And(x=w9115, y=w9116) -> (x .and. y?=w9114:bool)
                n3559 = Multiply(x=w9092, y=w9093) -> (x*y=w9048:dbl)
                n3560 = case shown="True" w9051 {
                  tunnel: [FALSE w9137] -> w9103
                  tunnel: w9101 -> [_ w9136]
                  tunnel: w9050 -> [_ w9135]
                  tunnel: w9028 -> [_ w9134]
                  frame False {
                  }
                  frame True {
                    n3561 = case shown="0" w9135 {
                      tunnel: [w9149 w9162 w9175 w9188 FALSE] -> w9137
                      tunnel: w9136 -> [w9148 w9161 w9174 w9187 _]
                      tunnel: w9134 -> [w9138 w9151 w9164 w9177 _]
                      frame 0 {
                        n3562 = Add(x=w9138, y=w9148) -> (x+y=w9146:sgl)
                        n3563 = Subtract(x=w9148, y=w9138) -> (x-y=w9142:sgl)
                        n3564 = To Single Precision Float(number=w9146) -> (single precision float=w9140:sgl)
                        n3565 = To Single Precision Float(number=w9142) -> (single precision float=w9141:sgl)
                        n3566 = local read "Specimen I high limit array"() -> (w9147:sgl[])
                        n3567 = local read "Specimen I (nA)"() -> (w9139:sgl)
                        n3568 = local read "Specimen I low limit array"() -> (w9143:sgl[])
                        n3569 = In Range and Coerce(upper limit=w9140, x=w9139, lower limit=w9141) -> (In Range?=w9150:bool)  [unwired: 1 out]
                        n3570 = Build Array (concatenate)(w9147, w9140) -> (w9145:sgl[])
                        n3571 = Build Array (concatenate)(w9143, w9141) -> (w9144:sgl[])
                        n3572 = Not(x=w9150) -> (.not. x?=w9149:bool)
                        n3573 = local write "Specimen I high limit array"(w9145) -> ()
                        n3574 = local write "Specimen I low limit array"(w9144) -> ()
                      }
                      frame 1 {
                        n3575 = Add(x=w9151, y=w9161) -> (x+y=w9159:sgl)
                        n3576 = Subtract(x=w9161, y=w9151) -> (x-y=w9155:sgl)
                        n3577 = To Single Precision Float(number=w9159) -> (single precision float=w9153:sgl)
                        n3578 = To Single Precision Float(number=w9155) -> (single precision float=w9154:sgl)
